vi "M19 Oxygen Concentrator Testbench.vi"() -> ()   [LabVIEW 2020]
uses:
  <vilib>/MakerHub/LINX/Public/Peripherals/Digital/Digital Write 1 Chan.vi
  <vilib>/MakerHub/LINX/Public/Peripherals/Digital/Digital Write N Chans.vi
  <vilib>/MakerHub/LINX/Private/Local IO/LinxDigitalWrite.vi
  <vilib>/MakerHub/LINX/Public/Utilities/Check Channel.vi
  <vilib>/MakerHub/LINX/Public/Utilities/Open Serial.vi
  <vilib>/MakerHub/LINX/Private/Utilties/Generate Error.vi
  <vilib>/MakerHub/LINX/LMH-LINX.lvlib
panel:
  in  "?":enum32{"Instrument Panel", "Settings"}(tab)
  in  "Operation":bool
  out "Sieve A Valve":bool
  out "Sieve B Valve":bool
  out "Equilisation Valve":bool
  in  "Precharge":i32(knob)=700 scale=0.0..2000.0
  in  "Seive A Valve":bool
  in  "Seive B Valve":bool
  in  "Equilize Valve":bool
  out "Active LOW/HIGH":bool
  in  "Sieve Charge / Sieve Purge":i32(knob)=4000 scale=0.0..10000.0
  in  "Sieve Charge / Sieve  Flush":i32(knob)=400 scale=0.0..2000.0
  in  "ON/OFF Switch":bool=TRUE
  out "Oxygen":cluster{dbl, i16, i16, i16}(graph)
  out "Oxygen %":dbl
  out "Oxygen mV":dbl
  in  "Compressor ON/OFF":bool
  in  "Input Pressure":dbl
  out "Loop Rate (Hz)":u32
  in  "Active LOW/HIGH":bool
  in  "O2 Ref %":dbl=98.5
  in  "mV at atm":dbl=14.0
  in  "mV at O2 Ref %":dbl=70.0
  in  "Equilization Valve DO Pin":u8=5
  in  "Sieve B Valve DO Pin":u8=6
  in  "Compressor Pin":u8=5
  in  "Sieve A Valve DO Pin":u8=4
  in  "Serial Port":refnum<visa-resource-name>="COM5"
  # "OFF"
  # "ON"
  # "%"
  # "Manual Valve Control"
  # "ON"
  # "ON"
  # "Auto"
  # "Manual"
  # "OFF"
  # "OFF"
  # "https://fracktal.in/"
  # "Source & Instructions : https://github.com/FracktalWorks/M19-oxygen-concentrator-testbench"
  # "Oxygen Sensor Calibration"
  # "Phisical Connnections:"
  # "Pin Declarations:"
  # "HIGH"
  # "LOW"
  # "Author: Vijay Raghav Varada\n               @vjvarada\n               vjvarada@fracktal.in"
  # "Publish Date: May 2021"
  # "https://github.com/FracktalWorks/M19-oxygen-concentrator-testbench/blob/main/LICENSE"
  # "https://fracktal.in/"
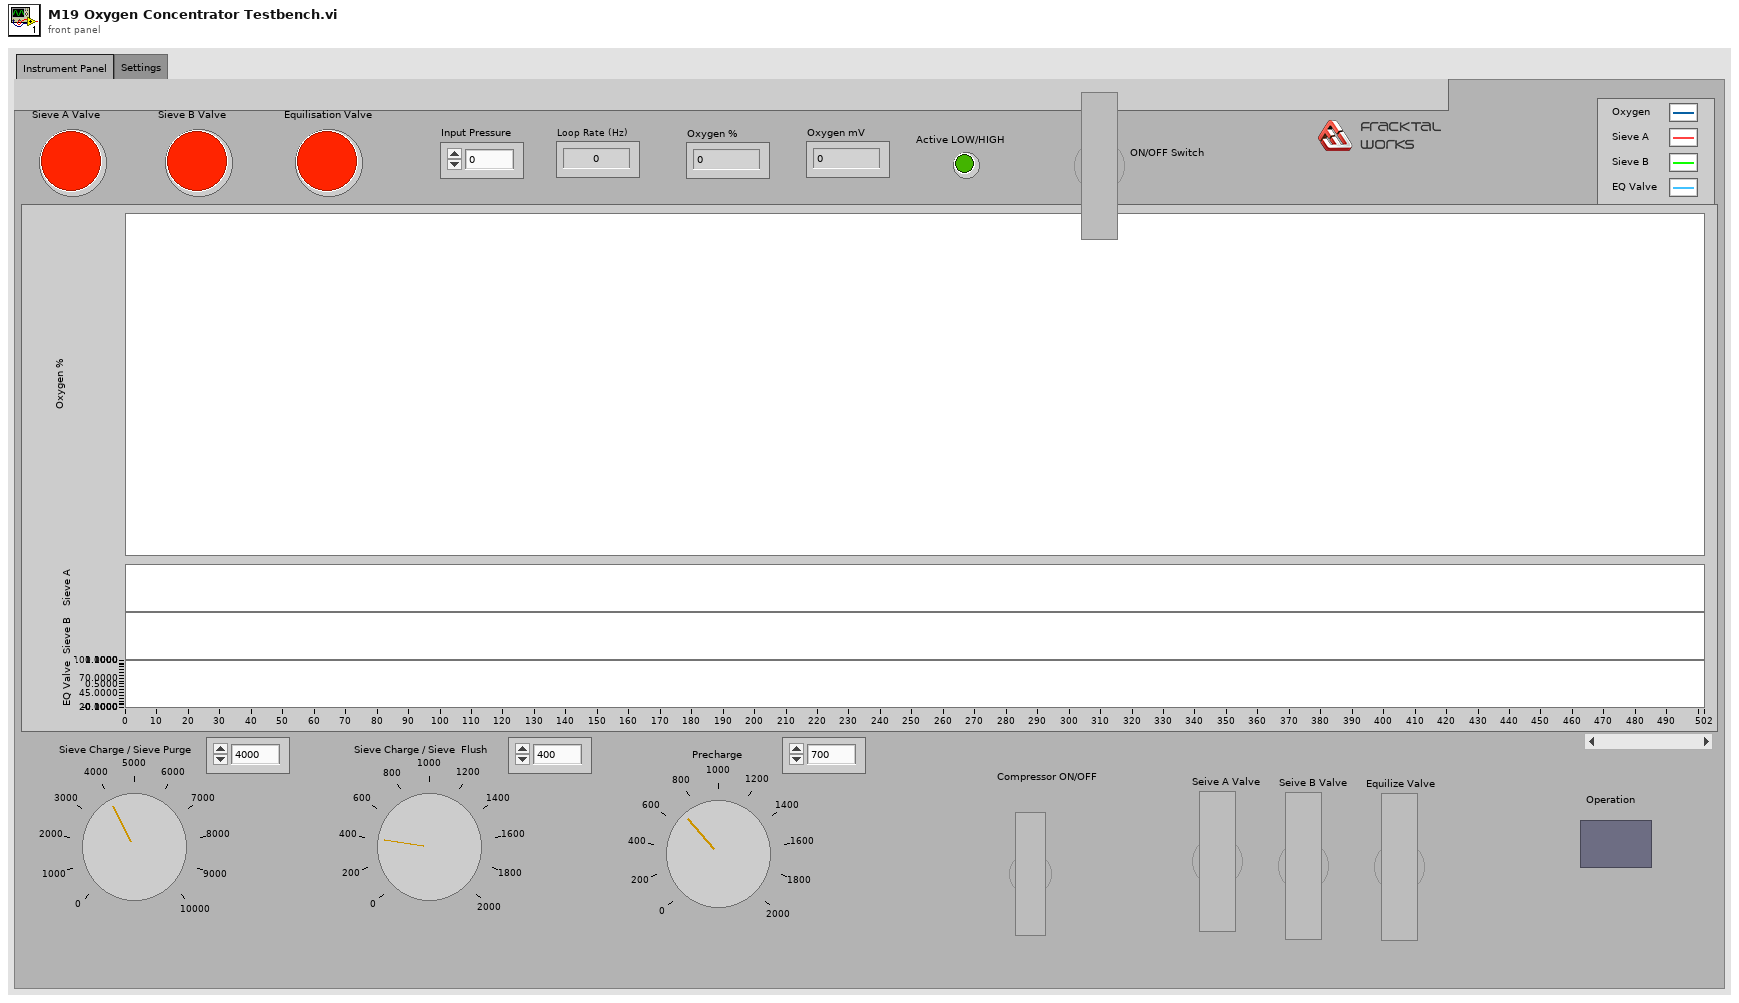
[diagram p1: front panel]
types:
  T1 = typedef "LMH-LINX.lvlib/LINX Ref.ctl" = cluster{"IO":T2, "Interface":T3, "LINX Device Config":T4}
  T2 = typedef "LMH-LINX.lvlib/Platform.ctl" = enum16{"Remote", "Local"}
  T3 = typedef "LMH-LINX.lvlib/Interface.ctl" = enum16{"Serial", "TCP"}
  T4 = typedef "LMH-LINX.lvlib/Device.lvlib/LINX Device Config.ctl" = cluster{"Interface":T3, "COM Port":refnum<visa-resource-name>, "TCP Configuration":T5, "Device Family":u8, "Device ID":u8, "Device Name":string, "TCP Ref":refnum<k5>, "Channels":T6}
  T5 = typedef "LMH-LINX.lvlib/Device.lvlib/TCP Config.ctl" = cluster{"IP Address":string, "Port":u16}
  T6 = typedef "LMH-LINX.lvlib/Channels.ctl" = cluster{"DI":u8[], "DO":u8[], "AI":u8[], "AO":u8[], "PWM":u8[], "QE":u8[], "UART":u8[], "I2C 2":u8[], "SPI":u8[], "CAN":u8[], "Servo":u8[], "AI Ref (V)":dbl, "AI Resolution (Bits)":u8, "AO Ref (V)":dbl, "AO Resolution (Bits)":u8}
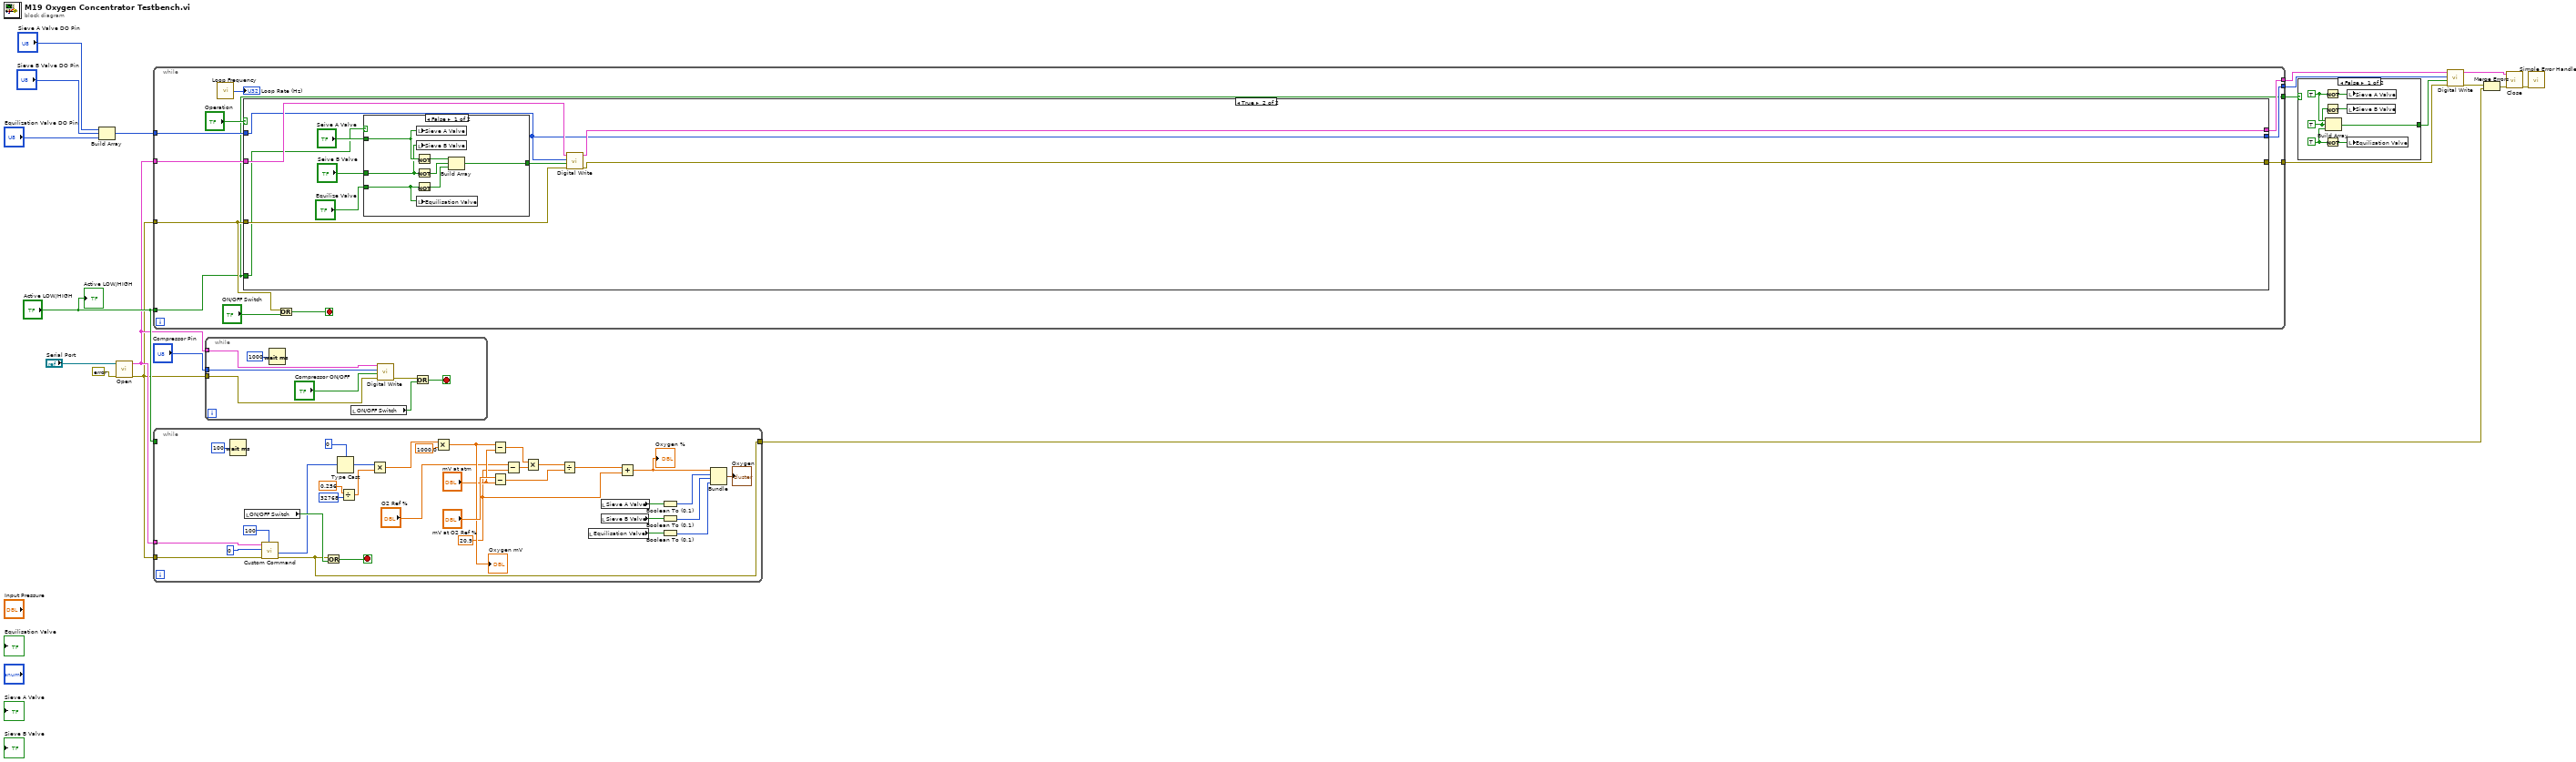
[diagram p0: block diagram]
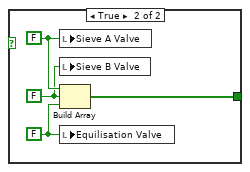
[diagram p2: hidden frame]
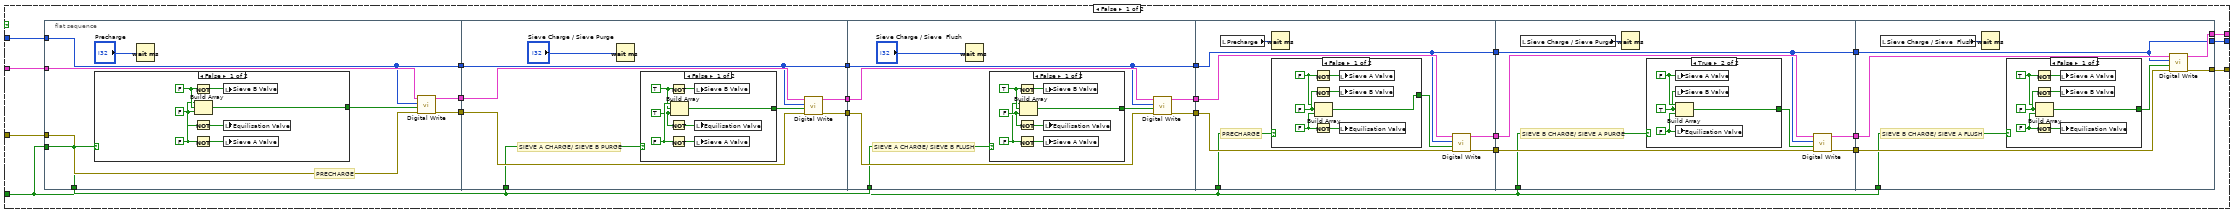
[diagram p3: hidden frame]
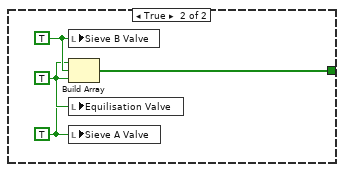
[diagram p4: hidden frame]
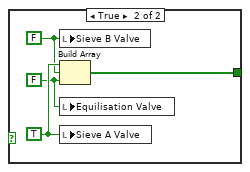
[diagram p5: hidden frame]
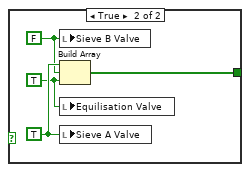
[diagram p6: hidden frame]
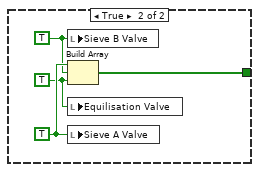
[diagram p7: hidden frame]
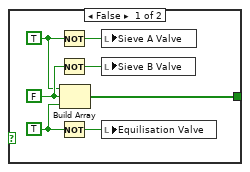
[diagram p8: hidden frame]
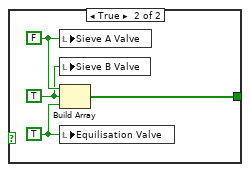
[diagram p9: hidden frame]
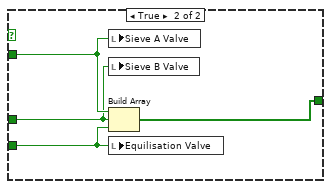
[diagram p10: hidden frame]
diagram:
  n1 = Build Array("Sieve A Valve DO Pin", "Sieve B Valve DO Pin", "Equilization Valve DO Pin") -> (w16:u8[])
  n2 = call-poly <vilib>:"Open.vi"("Error In"=errorcluster {"status"=FALSE, "code"=0, "source"=""}, "Serial Port"="Serial Port") -> ("Error Out"=w1:errorcluster, "LINX Resource"=w3:T1)  [unwired: 7 in, 1 out]
  n3 = while {
    tunnel: w3 -> [w30]
    tunnel: w1 -> [w23]
    tunnel: [w29] -> w9
    tunnel: [w26] -> w10
    tunnel: w16 -> [w28]
    tunnel: [w22] -> w8
    tunnel: [w21] -> w7
    tunnel: "Active LOW/HIGH" -> [w21]
    stop <- w24 stop-if-true
    n4 = call <vilib>:"Loop Frequency.vi"() -> ("Loop Rate (Hz)"=→"Loop Rate (Hz)":u32)
    n5 = case shown="True" "Operation" {
      tunnel: w23 -> [w54 w177]
      tunnel: w30 -> [w53 w178]
      tunnel: [w42 w176] -> w29
      tunnel: [w41 w175] -> w26
      tunnel: w28 -> [w40 w174]
      tunnel: [w34 w174] -> w22
      tunnel: w21 -> [w32 w169]
      frame False {
        n6 = flat-sequence {
          tunnel: w54 -> [w62]
          tunnel: w53 -> [w61]
          tunnel: [w60] -> w52
          tunnel: [w59] -> w51
          tunnel: w40 -> [w58]
          tunnel: [w58] -> w39
          tunnel: [w55] -> w33
          tunnel: w32 -> [w55]
          tunnel: w52 -> [w81]
          tunnel: w51 -> [w80]
          tunnel: [w79] -> w50
          tunnel: [w78] -> w49
          tunnel: w39 -> [w77]
          tunnel: [w77] -> w38
          tunnel: w33 -> [w74]
          tunnel: w50 -> [w100]
          tunnel: w49 -> [w99]
          tunnel: [w98] -> w48
          tunnel: [w97] -> w47
          tunnel: w38 -> [w96]
          tunnel: [w96] -> w37
          tunnel: w33 -> [w93]
          tunnel: w48 -> [w119]
          tunnel: w47 -> [w118]
          tunnel: [w117] -> w45
          tunnel: [w116] -> w44
          tunnel: w37 -> [w115]
          tunnel: [w115] -> w36
          tunnel: w32 -> [w112]
          tunnel: [w138] -> w46
          tunnel: w45 -> [w137]
          tunnel: w44 -> [w136]
          tunnel: [w135] -> w43
          tunnel: w36 -> [w134]
          tunnel: [w134] -> w35
          tunnel: w32 -> [w131]
          tunnel: w46 -> [w157]
          tunnel: w43 -> [w156]
          tunnel: [w155] -> w42
          tunnel: [w154] -> w41
          tunnel: w35 -> [w152]
          tunnel: [w152] -> w34
          tunnel: w32 -> [w150]
          frame #0 {
            # "PRECHARGE"
            n7 = case shown="False" w55 {
              tunnel: [w64 w70] -> w56
              frame False {
                w66 = FALSE
                w67 = FALSE
                w65 = FALSE
                n8 = Not(x=w67) -> (.not. x?=w69:bool)
                n9 = Not(x=w66) -> (.not. x?=w63:bool)
                n10 = Not(x=w65) -> (.not. x?=w68:bool)
                n11 = Build Array(w65, w67, w66) -> (w64:bool[])
                n12 = local write "Sieve B Valve"(w69) -> ()
                n13 = local write "Equilisation Valve"(w63) -> ()
                n14 = local write "Sieve A Valve"(w68) -> ()
              }
              frame True {
                w72 = TRUE
                w73 = TRUE
                w71 = TRUE
                n15 = local write "Sieve B Valve"(w73) -> ()
                n16 = Build Array(w71, w73, w72) -> (w70:bool[])
                n17 = local write "Equilisation Valve"(w72) -> ()
                n18 = local write "Sieve A Valve"(w71) -> ()
              }
            }
            n19 = Wait (ms)(milliseconds to wait="Precharge") -> ()  [unwired: 1 out]
            n20 = call-poly <vilib>:"Digital Write.vi"("Error In"=w62, "Values"=w56, "DO Channels"=w58, "LINX Resource"=w61) -> ("Error Out"=w59:errorcluster, "LINX Resource"=w60:T1)  [unwired: 6 in]
          }
          frame #1 {
            # "SIEVE A CHARGE/ SIEVE B PURGE"
            n21 = Wait (ms)(milliseconds to wait="Sieve Charge / Sieve Purge") -> ()  [unwired: 1 out]
            n22 = case shown="False" w74 {
              tunnel: [w88 w89] -> w75
              frame False {
                w85 = TRUE
                w86 = TRUE
                w87 = FALSE
                n23 = Not(x=w86) -> (.not. x?=w83:bool)
                n24 = Not(x=w85) -> (.not. x?=w82:bool)
                n25 = Not(x=w87) -> (.not. x?=w84:bool)
                n26 = Build Array(w87, w86, w85) -> (w88:bool[])
                n27 = local write "Sieve B Valve"(w83) -> ()
                n28 = local write "Equilisation Valve"(w82) -> ()
                n29 = local write "Sieve A Valve"(w84) -> ()
              }
              frame True {
                w90 = FALSE
                w91 = FALSE
                w92 = TRUE
                n30 = local write "Sieve B Valve"(w91) -> ()
                n31 = Build Array(w92, w91, w90) -> (w89:bool[])
                n32 = local write "Equilisation Valve"(w90) -> ()
                n33 = local write "Sieve A Valve"(w92) -> ()
              }
            }
            n34 = call-poly <vilib>:"Digital Write.vi"("Error In"=w80, "Values"=w75, "DO Channels"=w77, "LINX Resource"=w81) -> ("Error Out"=w78:errorcluster, "LINX Resource"=w79:T1)  [unwired: 6 in]
          }
          frame #2 {
            # "SIEVE A CHARGE/ SIEVE B FLUSH"
            n35 = Wait (ms)(milliseconds to wait="Sieve Charge / Sieve  Flush") -> ()  [unwired: 1 out]
            n36 = case shown="False" w93 {
              tunnel: [w101 w108] -> w94
              frame False {
                w103 = FALSE
                w104 = TRUE
                w102 = FALSE
                n37 = Not(x=w104) -> (.not. x?=w107:bool)
                n38 = Not(x=w103) -> (.not. x?=w106:bool)
                n39 = Not(x=w102) -> (.not. x?=w105:bool)
                n40 = Build Array(w102, w104, w103) -> (w101:bool[])
                n41 = local write "Sieve B Valve"(w107) -> ()
                n42 = local write "Equilisation Valve"(w106) -> ()
                n43 = local write "Sieve A Valve"(w105) -> ()
              }
              frame True {
                w109 = TRUE
                w110 = FALSE
                w111 = TRUE
                n44 = local write "Sieve B Valve"(w110) -> ()
                n45 = Build Array(w111, w110, w109) -> (w108:bool[])
                n46 = local write "Equilisation Valve"(w109) -> ()
                n47 = local write "Sieve A Valve"(w111) -> ()
              }
            }
            n48 = call-poly <vilib>:"Digital Write.vi"("Error In"=w99, "Values"=w94, "DO Channels"=w96, "LINX Resource"=w100) -> ("Error Out"=w97:errorcluster, "LINX Resource"=w98:T1)  [unwired: 6 in]
          }
          frame #3 {
            # "PRECHARGE"
            n49 = local read "Precharge"() -> (w114:i32)
            n50 = Wait (ms)(milliseconds to wait=w114) -> ()  [unwired: 1 out]
            n51 = case shown="False" w112 {
              tunnel: [w121 w127] -> w113
              frame False {
                w123 = FALSE
                w124 = FALSE
                w122 = FALSE
                n52 = Not(x=w122) -> (.not. x?=w125:bool)
                n53 = Not(x=w124) -> (.not. x?=w120:bool)
                n54 = Not(x=w123) -> (.not. x?=w126:bool)
                n55 = Build Array(w122, w124, w123) -> (w121:bool[])
                n56 = local write "Sieve A Valve"(w125) -> ()
                n57 = local write "Sieve B Valve"(w120) -> ()
                n58 = local write "Equilisation Valve"(w126) -> ()
              }
              frame True {
                w128 = TRUE
                w129 = TRUE
                w130 = TRUE
                n59 = local write "Sieve B Valve"(w129) -> ()
                n60 = Build Array(w130, w129, w128) -> (w127:bool[])
                n61 = local write "Equilisation Valve"(w128) -> ()
                n62 = local write "Sieve A Valve"(w130) -> ()
              }
            }
            n63 = call-poly <vilib>:"Digital Write.vi"("Error In"=w118, "Values"=w113, "DO Channels"=w115, "LINX Resource"=w119) -> ("Error Out"=w116:errorcluster, "LINX Resource"=w117:T1)  [unwired: 6 in]
          }
          frame #4 {
            # "SIEVE B CHARGE/ SIEVE A PURGE"
            n64 = local read "Sieve Charge / Sieve Purge"() -> (w133:i32)
            n65 = Wait (ms)(milliseconds to wait=w133) -> ()  [unwired: 1 out]
            n66 = case shown="True" w131 {
              tunnel: [w140 w146] -> w132
              frame False {
                w141 = TRUE
                w143 = FALSE
                w142 = TRUE
                n67 = Not(x=w142) -> (.not. x?=w144:bool)
                n68 = Not(x=w143) -> (.not. x?=w145:bool)
                n69 = Not(x=w141) -> (.not. x?=w139:bool)
                n70 = Build Array(w142, w143, w141) -> (w140:bool[])
                n71 = local write "Sieve A Valve"(w144) -> ()
                n72 = local write "Sieve B Valve"(w145) -> ()
                n73 = local write "Equilisation Valve"(w139) -> ()
              }
              frame True {
                w148 = FALSE
                w147 = TRUE
                w149 = FALSE
                n74 = local write "Sieve A Valve"(w149) -> ()
                n75 = local write "Sieve B Valve"(w147) -> ()
                n76 = Build Array(w149, w147, w148) -> (w146:bool[])
                n77 = local write "Equilisation Valve"(w148) -> ()
              }
            }
            n78 = call-poly <vilib>:"Digital Write.vi"("Error In"=w136, "Values"=w132, "DO Channels"=w134, "LINX Resource"=w137) -> ("Error Out"=w135:errorcluster, "LINX Resource"=w138:T1)  [unwired: 6 in]
          }
          frame #5 {
            # "SIEVE B CHARGE/ SIEVE A FLUSH"
            n79 = local read "Sieve Charge / Sieve  Flush"() -> (w153:i32)
            n80 = Wait (ms)(milliseconds to wait=w153) -> ()  [unwired: 1 out]
            n81 = case shown="False" w150 {
              tunnel: [w158 w165] -> w151
              frame False {
                w161 = FALSE
                w160 = FALSE
                w159 = TRUE
                n82 = Not(x=w159) -> (.not. x?=w162:bool)
                n83 = Not(x=w160) -> (.not. x?=w163:bool)
                n84 = Not(x=w161) -> (.not. x?=w164:bool)
                n85 = Build Array(w159, w160, w161) -> (w158:bool[])
                n86 = local write "Sieve A Valve"(w162) -> ()
                n87 = local write "Sieve B Valve"(w163) -> ()
                n88 = local write "Equilisation Valve"(w164) -> ()
              }
              frame True {
                w166 = TRUE
                w167 = TRUE
                w168 = FALSE
                n89 = local write "Sieve A Valve"(w168) -> ()
                n90 = local write "Sieve B Valve"(w167) -> ()
                n91 = Build Array(w168, w167, w166) -> (w165:bool[])
                n92 = local write "Equilisation Valve"(w166) -> ()
              }
            }
            n93 = call-poly <vilib>:"Digital Write.vi"("Error In"=w156, "Values"=w151, "DO Channels"=w152, "LINX Resource"=w157) -> ("Error Out"=w154:errorcluster, "LINX Resource"=w155:T1)  [unwired: 6 in]
          }
        }
      }
      frame True {
        n94 = case shown="False" w169 {
          tunnel: [w185 w189] -> w173
          tunnel: "Seive A Valve" -> [w181 w188]
          tunnel: "Seive B Valve" -> [w180 w187]
          tunnel: "Equilize Valve" -> [w179 w186]
          frame False {
            n95 = Not(x=w181) -> (.not. x?=w182:bool)
            n96 = Not(x=w180) -> (.not. x?=w183:bool)
            n97 = Not(x=w179) -> (.not. x?=w184:bool)
            n98 = local write "Sieve A Valve"(w181) -> ()
            n99 = local write "Sieve B Valve"(w180) -> ()
            n100 = local write "Equilisation Valve"(w179) -> ()
            n101 = Build Array(w182, w183, w184) -> (w185:bool[])
          }
          frame True {
            n102 = local write "Sieve A Valve"(w188) -> ()
            n103 = local write "Sieve B Valve"(w187) -> ()
            n104 = Build Array(w188, w187, w186) -> (w189:bool[])
            n105 = local write "Equilisation Valve"(w186) -> ()
          }
        }
        n106 = call-poly <vilib>:"Digital Write.vi"("Error In"=w177, "Values"=w173, "DO Channels"=w174, "LINX Resource"=w178) -> ("Error Out"=w175:errorcluster, "LINX Resource"=w176:T1)  [unwired: 6 in]
      }
    }
    n107 = Or(x=w23, y="ON/OFF Switch") -> (x .or. y?=w24:bool)
  }
  n108 = while {
    tunnel: w1 -> [w220]
    tunnel: w3 -> [w221]
    tunnel: [w194] -> w4
    tunnel: "Active LOW/HIGH" -> [_]
    stop <- w222 stop-if-true
    w201 = 20.9 ("y")
    n109 = Wait (ms)(milliseconds to wait=u32 100) -> ()  [unwired: 1 out]
    n110 = local read "ON/OFF Switch"() -> (w223:bool)
    n111 = call <vilib>:"Custom Command.vi"("Timeout (100 ms)"=100, "Error In"=w220, "Custom Command Number"=u16 0, "LINX Resource"=w221) -> ("Error Out"=w194:errorcluster, "Response"=w217:u8[])  [unwired: 4 in, 2 out]
    n112 = Or(x=w194, y=w223) -> (x .or. y?=w222:bool)
    n113 = Type Cast(type=u16 0, x=w217) -> (*(type *) &x=w215:u16)
    n114 = Divide(x=0.256, y=u16 32768) -> (x/y=w213:dbl)
    n115 = Multiply(x=w215, y=w213) -> (x*y=w207:dbl)
    n116 = Multiply(x=w207, y=1000.0) -> (x*y=w205:dbl)
    "Oxygen mV" <- w205
    n117 = Subtract(x=w205, y="mV at atm") -> (x-y=w211:dbl)
    n118 = Subtract(x="mV at O2 Ref %", y="mV at atm") -> (x-y=w204:dbl)
    n119 = Subtract(x="O2 Ref %", y=w201) -> (x-y=w210:dbl)
    n120 = Multiply(x=w211, y=w210) -> (x*y=w209:dbl)
    n121 = Divide(x=w209, y=w204) -> (x/y=w202:dbl)
    n122 = local read "Equilisation Valve"() -> (w191:bool)
    n123 = local read "Sieve A Valve"() -> (w193:bool)
    n124 = local read "Sieve B Valve"() -> (w192:bool)
    n125 = Add(x=w202, y=w201) -> (x+y=w199:dbl)
    "Oxygen %" <- w199
    n126 = Boolean To (0,1)(Boolean=w193) -> (0, 1=w196:i16)
    n127 = Boolean To (0,1)(Boolean=w192) -> (0, 1=w197:i16)
    n128 = Boolean To (0,1)(Boolean=w191) -> (0, 1=w198:i16)
    n129 = Bundle(w199, w196, w197, w198) -> (→"Oxygen":cluster{dbl, i16, i16, i16})  [unwired: 1 in]
  }
  n130 = while {
    tunnel: w3 -> [w231]
    tunnel: "Compressor Pin" -> [w230]
    tunnel: w1 -> [w228]
    stop <- w224 stop-if-true
    n131 = Wait (ms)(milliseconds to wait=u32 1000) -> ()  [unwired: 1 out]
    n132 = local read "ON/OFF Switch"() -> (w226:bool)
    n133 = call-poly <vilib>:"Digital Write.vi"("Error In"=w228, "Output Value"="Compressor ON/OFF", "DO Channel"=w230, "LINX Resource"=w231) -> ("Error Out"=w225:errorcluster)  [unwired: 6 in, 1 out]
    n134 = Or(x=w225, y=w226) -> (x .or. y?=w224:bool)
  }
  n135 = case shown="False" w7 {
    tunnel: [w232 w242] -> w6
    frame False {
      w234 = TRUE
      w233 = TRUE
      w235 = TRUE
      n136 = Not(x=w235) -> (.not. x?=w237:bool)
      n137 = Not(x=w233) -> (.not. x?=w238:bool)
      n138 = Not(x=w234) -> (.not. x?=w236:bool)
      n139 = Build Array(w235, w233, w234) -> (w232:bool[])
      n140 = local write "Sieve A Valve"(w237) -> ()
      n141 = local write "Sieve B Valve"(w238) -> ()
      n142 = local write "Equilisation Valve"(w236) -> ()
    }
    frame True {
      w239 = FALSE
      w241 = FALSE
      w240 = FALSE
      n143 = local write "Sieve A Valve"(w241) -> ()
      n144 = local write "Sieve B Valve"(w240) -> ()
      n145 = Build Array(w241, w240, w239) -> (w242:bool[])
      n146 = local write "Equilisation Valve"(w239) -> ()
    }
  }
  n147 = call-poly <vilib>:"Digital Write.vi"("Error In"=w10, "Values"=w6, "DO Channels"=w8, "LINX Resource"=w9) -> ("Error Out"=w11:errorcluster, "LINX Resource"=w12:T1)  [unwired: 6 in]
  n148 = Merge Errors(w11, w4) -> (w17:errorcluster)
  n149 = call <vilib>:"Close.vi"("Error In"=w17, "LINX Resource"=w12) -> ("Error Out"=w20:errorcluster)  [unwired: 9 in]
  n150 = call <vilib>:"Simple Error Handler.vi"("error in (no error)"=w20) -> ()  [unwired: 4 in, 5 out]
  "Active LOW/HIGH" <- "Active LOW/HIGH"
